vi "Finding Center.vi"() -> ()   [LabVIEW 2014]
panel:
  out "x+y":cluster{"X":sgl, "Y":sgl}
  out "XY Graph":cluster{"X":sgl, "Y":sgl}[](graph)
  out "array":sgl[](array[numeric])
  in  "Bound Region":T1
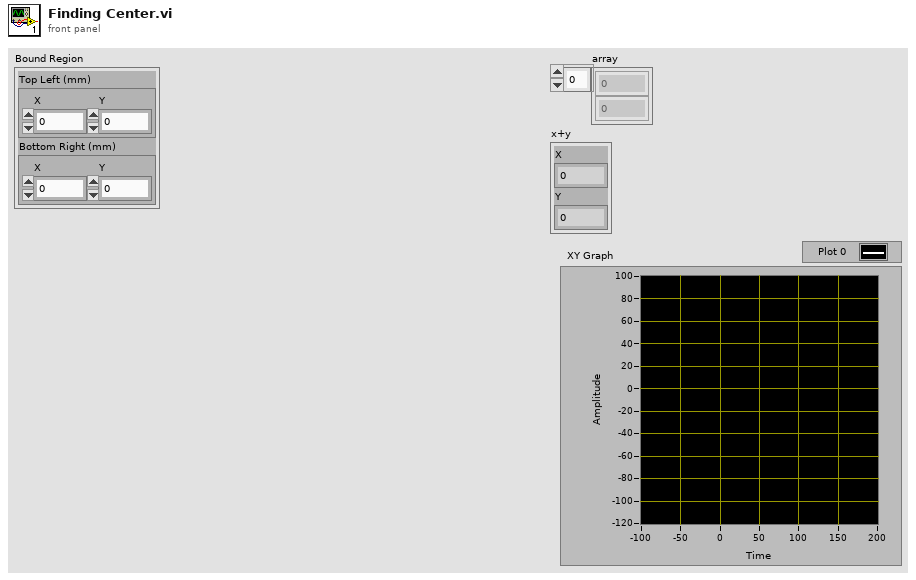
[diagram p1: front panel]
types:
  T1 = cluster{"Top Left (mm)":cluster{"X":sgl, "Y":sgl}, "Bottom Right (mm)":cluster{"X":sgl, "Y":sgl}}
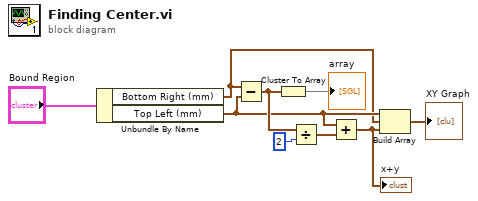
[diagram p0: block diagram]
diagram:
  n1 = Unbundle By Name("Bound Region") -> ("Bottom Right (mm)"=w1:cluster{"X":sgl, "Y":sgl}, "Top Left (mm)"=w4:cluster{"X":sgl, "Y":sgl})
  n2 = Subtract(x=w1, y=w4) -> (x-y=w6:cluster{"X":sgl, "Y":sgl})
  n3 = Cluster To Array(cluster=w6) -> (array=→"array":sgl[])
  n4 = Divide(x=w6, y=2) -> (x/y=w5:cluster{"X":sgl, "Y":sgl})
  n5 = Add(x=w4, y=w5) -> (x+y=w3:cluster{"X":sgl, "Y":sgl})
  "x+y" <- w3
  n6 = Build Array(w4, w1, w3) -> (→"XY Graph":cluster{"X":sgl, "Y":sgl}[])
